vi "FallingEdge.vi"(11 "BooleanIn":bool=TRUE) -> (3 "BooleanOut":bool)   [LabVIEW 2012]
doc: "Outputs true only if the previous instance of BooleanIn is true and the current instance of BooleanIn is false, otherwise outputs false (the first call to this VI will always return false)."
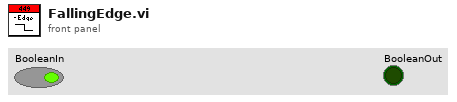
[diagram p1: front panel]
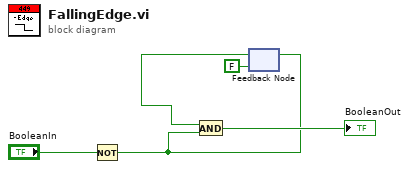
[diagram p0: block diagram]
diagram:
  n1 = Not(x="BooleanIn") -> (.not. x?=w2:bool)
  n2 = feedback-in #1(w2) -> ()
  n3 = feedback #1(FALSE ("BooleanIn")) -> (w1:bool)
  n4 = And(x=w1, y=w2) -> (x .and. y?=→"BooleanOut":bool)
